vi "DisposeAdsResources.vi"(8 "error in (no error)":errorcluster, 11 "AdsNET in":refnum<class "AdsNET.lvclass">) -> (0 "error out":errorcluster, 3 "AdsNET out":refnum<class "AdsNET.lvclass">)   [LabVIEW 2016, in "TCatAdsNet.lvlib" / "AdsNET.lvclass"]
doc: "Releases the resources used by TcAdsClient."
uses:
  AdsNET.lvclass
  AdsNET.lvclass/AdsNET.ctl
  C:/Users/Maurizio/Projects/sentiero-beckoff/DLL/TwinCAT.Ads.dll
  sentiero-beckoff/DLL/TwinCAT.Ads.dll
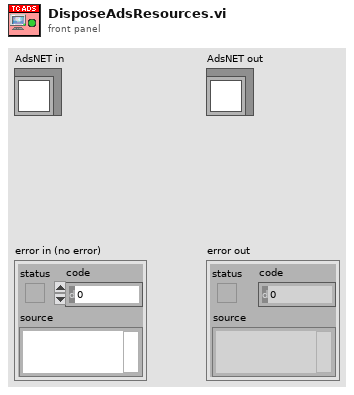
[diagram p1: front panel]
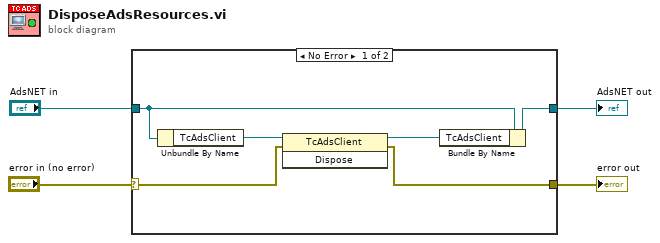
[diagram p0: block diagram]
diagram:
  n1 = case shown="No Error" "error in (no error)" {
    selector: "error in (no error)" -> [w6 w12]
    tunnel: [w5 w12] -> w3
    tunnel: [w8 w11] -> w1
    tunnel: "AdsNET in" -> [w10 w11]
    frame No Error {
      n2 = Unbundle By Name(w10) -> ("TcAdsClient"=w9:refnum<k24>)
      n3 = invoke class="TcAdsClient" method="Dispose"(reference=w9, error in=w6) -> (reference out=w7:refnum<k24>, error out=w5:errorcluster)  [unwired: 1 in, 1 out]
      n4 = Bundle By Name(cluster=w10, "TcAdsClient"=w7) -> (w8:refnum<class "AdsNET.lvclass">)
    }
    frame Error {
    }
  }
  "error out" <- w3
  "AdsNET out" <- w1
